vi "23384_Davis_Poku_Amankwa_Amankwa.DavisPoku.MNE1201.7.4_348263_351171658.vi"() -> ()   [LabVIEW 2018]
panel:
  out "Divided by 0?":bool
  out "Result":dbl
  in  "Y":dbl
  in  "X":dbl
  in  "Operation":T1(ring)
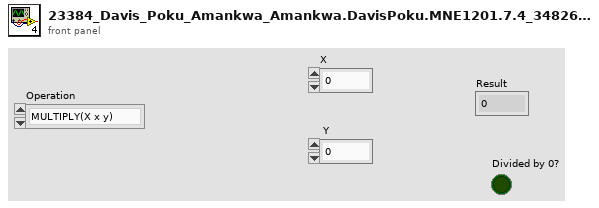
[diagram p1: front panel]
types:
  T1 = enum16{"MULTIPLY(X x y)", "DIVIDE(X/Y)", "SUBSTRACT(X-Y)", "ADD(X+Y)"}
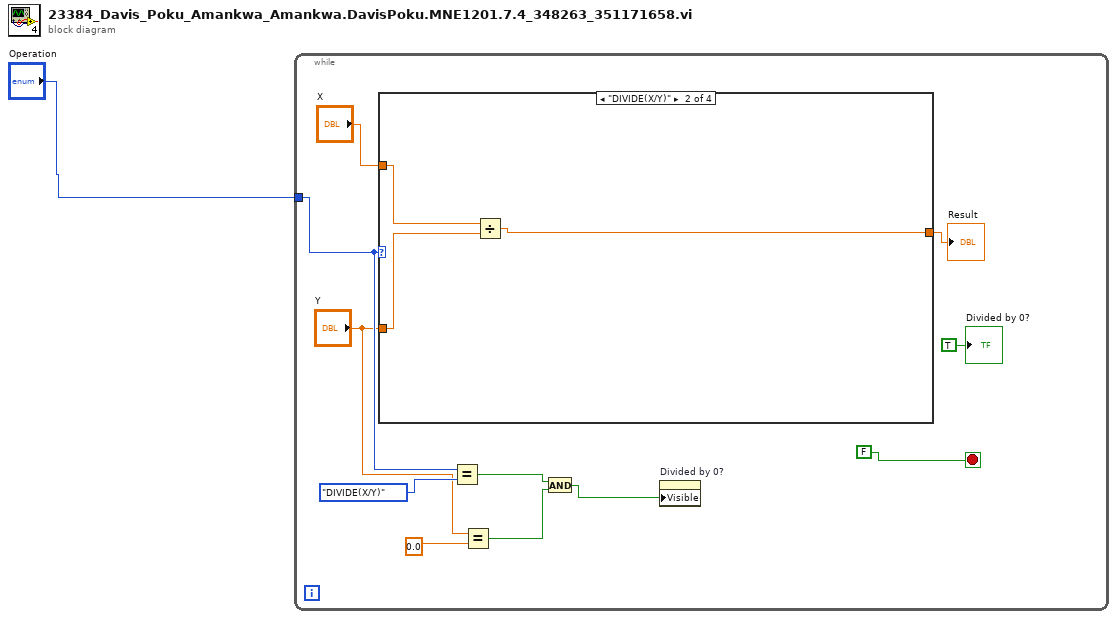
[diagram p0: block diagram]
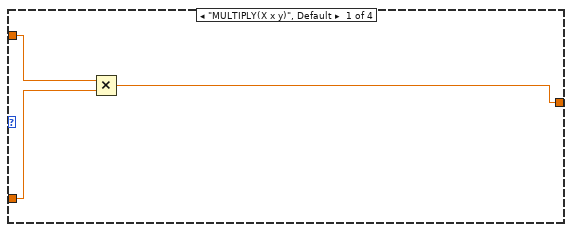
[diagram p2: hidden frame]
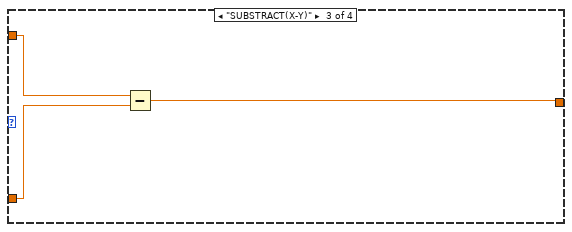
[diagram p3: hidden frame]
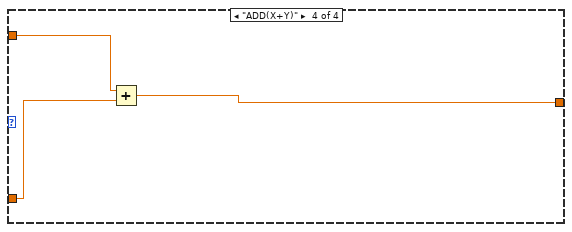
[diagram p4: hidden frame]
diagram:
  n1 = while {
    tunnel: "Operation" -> [w8]
    stop <- FALSE stop-if-true
    n2 = case shown="\"DIVIDE(X/Y)\"" w8 {
      tunnel: "X" -> [w15 w18 w21 w23]
      tunnel: "Y" -> [w14 w16 w20 w24]
      tunnel: [w13 w17 w19 w22] -> w11
      frame "MULTIPLY(X x y)", Default {
        n3 = Multiply(x=w15, y=w14) -> (x*y=w13:dbl)
      }
      frame "DIVIDE(X/Y)" {
        n4 = Divide(x=w18, y=w16) -> (x/y=w17:dbl)
      }
      frame "SUBSTRACT(X-Y)" {
        n5 = Subtract(x=w21, y=w20) -> (x-y=w19:dbl)
      }
      frame "ADD(X+Y)" {
        n6 = Add(x=w23, y=w24) -> (x+y=w22:dbl)
      }
    }
    "Result" <- w11
    n7 = Equal?(x=w8, y=T1."DIVIDE(X/Y)" ("Operation")) -> (x = y?=w5:bool)
    n8 = Equal?(x="Y", y=0.0) -> (x = y?=w4:bool)
    n9 = And(x=w5, y=w4) -> (x .and. y?=w3:bool)
    n10 = property on="Divided by 0?" class="Bool (strict)"("Visible"=w3) -> ()  [unwired: 2 in, 2 out]
    "Divided by 0?" <- TRUE ("Divided by 0?")
  }
